vi "LINX - Interactions LED Matrix.vi"() -> ()   [LabVIEW 2019]
doc: "LED Matrix\n\nThis example demonstrates how to use the LED Matrix included in the LabVIEW Interactions Parts Kit. Make sure\nthat you are using the correct firmware version so the matrix functions are supported. \n\nInstructions:\n1. Select the COM Port associated with the LINX device\n2. Toggle the Smart Write to desired value\n3. Enter the 16 Channels connected to Matrix in the correct order\n4. Click the Run Arrow."
uses:
  <vilib>/MakerHub/LINX/Public/Utilities/Open Serial.vi
  <vilib>/MakerHub/LINX/LMH-LINX.lvlib
  <vilib>/MakerHub/LINX/Public/Sensors/Digilent/Interaction Parts Kit/Interaction Parts Kit.lvlib
panel:
  in  "Channels":T1
  in  "Display Type":enum8{"Matrix", "7 Segment"}(ring)
  in  "Smart Write? (T)":bool=TRUE
  out "Loop Rate (Hz)":u32
  in  "Stop Button":bool
  in  "LEDs to Light":bool[][](array[boolean])=[[TRUE, TRUE, TRUE, TRUE, TRUE, TRUE, TRUE, FALSE], [TRUE, TRUE, TRUE, TRUE, TRUE, TRUE, FALSE, FALSE], [TRUE, TRUE, TRUE, TRUE, TRUE, FALSE, FALSE, FALSE], [TRUE, TRUE, TRUE, TRUE, FALSE, FALSE, FALSE, FALSE], [TRUE, TRUE, TRUE, FALSE, FALSE, FALSE, FALSE, FALSE], [TRUE, TRUE, FALSE, FALSE, FALSE, FALSE, FALSE, FALSE], [TRUE, FALSE, FALSE, FALSE, FALSE, FALSE, FALSE, FALSE], [FALSE, FALSE, FALSE, FALSE, FALSE, FALSE, FALSE, TRUE]]
  in  "Serial Port":refnum<visa-resource-name>="N/A"
  # "LED Matrix\n\nThis example demonstrates how to use the LED Matrix included in the LabVIEW Interactions Parts Kit.  Make sure\nthat you are using the correct firmware version so the matrix functions are supported. \n\nInstructions:\n1. Select the COM Port associated with the LINX device\n2. Toggle the Smart Write to desired value\n3. Enter the 16 Channels connected to Matrix in the correct order\n4. Select \"Matrix\" under Display Type\n5. Click the Run Arrow."
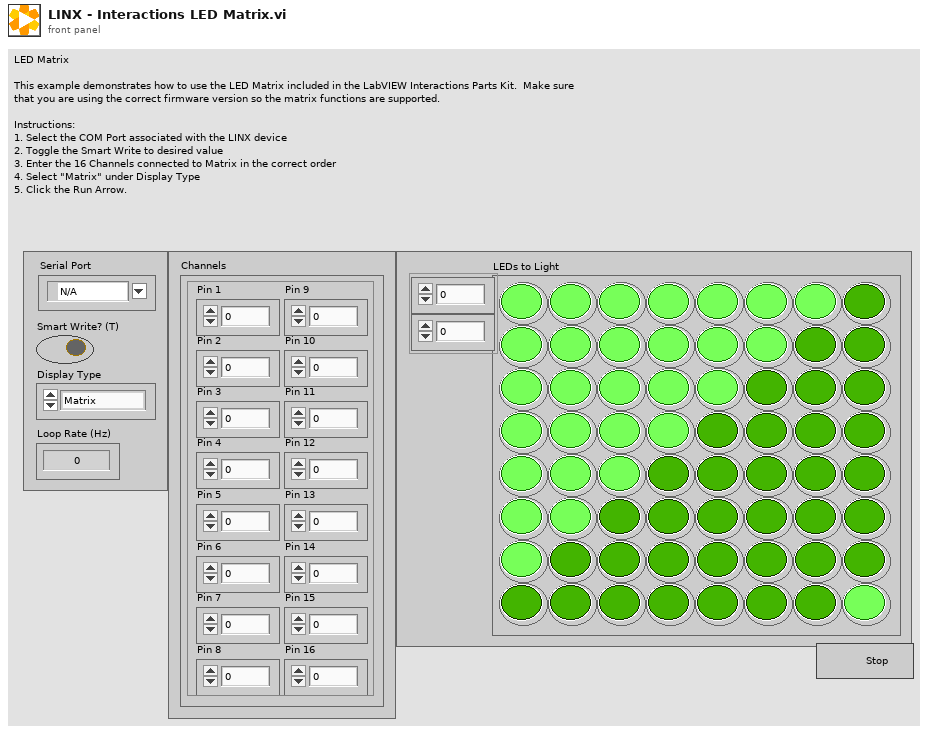
[diagram p1: front panel]
types:
  T1 = cluster{"Pin 1":u8, "Pin 2":u8, "Pin 3":u8, "Pin 4":u8, "Pin 5":u8, "Pin 6":u8, "Pin 7":u8, "Pin 8":u8, "Pin 9":u8, "Pin 10":u8, "Pin 11":u8, "Pin 12":u8, "Pin 13":u8, "Pin 14":u8, "Pin 15":u8, "Pin 16":u8}
  T2 = typedef "LMH-LINX.lvlib/LINX Ref.ctl" = cluster{"IO":T3, "Interface":T4, "LINX Device Config":T5}
  T3 = typedef "LMH-LINX.lvlib/Platform.ctl" = enum16{"Remote", "Local"}
  T4 = typedef "LMH-LINX.lvlib/Interface.ctl" = enum16{"Serial", "TCP"}
  T5 = typedef "LMH-LINX.lvlib/Device.lvlib/LINX Device Config.ctl" = cluster{"Interface":T4, "COM Port":refnum<visa-resource-name>, "TCP Configuration":T6, "Device Family":u8, "Device ID":u8, "Device Name":string, "TCP Ref":refnum<k5>, "Channels":T7}
  T6 = typedef "LMH-LINX.lvlib/Device.lvlib/TCP Config.ctl" = cluster{"IP Address":string, "Port":u16}
  T7 = typedef "LMH-LINX.lvlib/Channels.ctl" = cluster{"DI":u8[], "DO":u8[], "AI":u8[], "AO":u8[], "PWM":u8[], "QE":u8[], "UART":u8[], "I2C 2":u8[], "SPI":u8[], "CAN":u8[], "Servo":u8[], "AI Ref (V)":dbl, "AI Resolution (Bits)":u8, "AO Ref (V)":dbl, "AO Resolution (Bits)":u8}
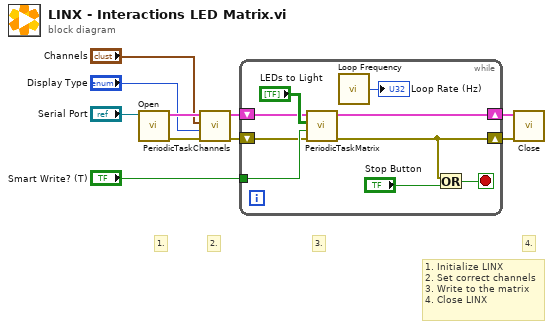
[diagram p0: block diagram]
diagram:
  # "1."
  # "2."
  # "3."
  # "4."
  # "1. Initialize LINX\n2. Set correct channels\n3. Write to the matrix\n4. Close LINX"
  n1 = call-poly <vilib>:"Open.vi"("Serial Port"="Serial Port") -> ("Error Out"=w9:errorcluster, "LINX Resource"=w10:T2)  [unwired: 8 in, 1 out]
  n2 = call <vilib>:"PeriodicTaskChannels.vi"("Error In"=w9, "Display Type"="Display Type", "Channels"="Channels", "LINX Resource"=w10) -> ("Error Out"=w6:errorcluster, "LINX Resource"=w7:T2)  [unwired: 4 in, 1 out]
  n3 = while {
    shift-right: [w18] -> w5
    shift-left: w7 -> [w15]
    shift-right: [w11] -> w4
    shift-left: w6 -> [w14]
    tunnel: "Smart Write? (T)" -> [w16]
    stop <- w13 stop-if-true
    n4 = call <vilib>:"PeriodicTaskMatrix.vi"("Error In"=w14, "Smart Write (T)?"=w16, "LEDs to Light"="LEDs to Light", "LINX Resource"=w15) -> ("Error Out"=w11:errorcluster, "LINX Resource"=w18:T2)  [unwired: 5 in, 1 out]
    n5 = call <vilib>:"Loop Frequency.vi"() -> ("Loop Rate (Hz)"=→"Loop Rate (Hz)":u32)
    n6 = Or(x=w11, y="Stop Button") -> (x .or. y?=w13:bool)
  }
  n7 = call <vilib>:"Close.vi"("Error In"=w4, "LINX Resource"=w5) -> ()  [unwired: 9 in, 1 out]
